vi "slscswitch Initialize.vi"(8 "error in (no error)":errorcluster, 9 "reset device (T)":bool, 11 "device":refnum<k21>) -> (0 "error out":errorcluster, 3 "SLSC Switch out":refnum<class "SLSC Switch.lvclass">)   [LabVIEW 2015, in "SLSC Switch.lvclass"]
uses:
  SLSC Switch.lvclass
  SLSC Switch.lvclass/SLSC Switch.ctl
  <vilib>/SLSC/Initialize Session without Resources.vi
  Route Manager/Route Manager.lvclass
  <vilib>/SLSC/SLSC.lvlib
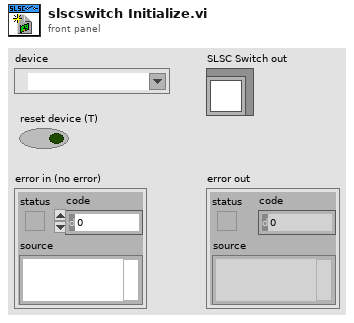
[diagram p1: front panel]
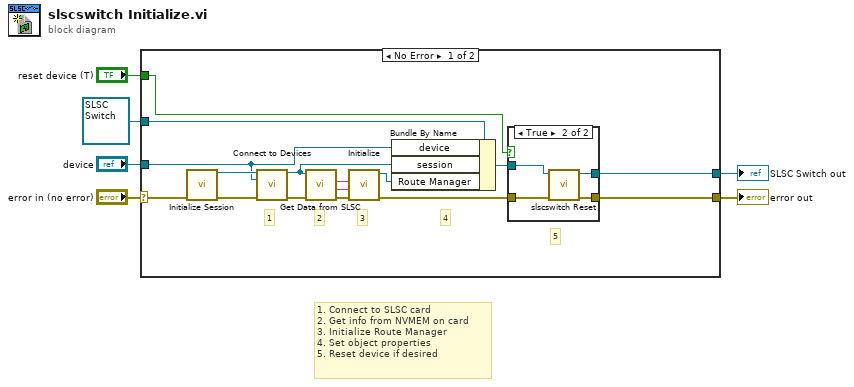
[diagram p0: block diagram]
diagram:
  # "1. Connect to SLSC card\n2. Get info from NVMEM on card\n3. Initialize Route Manager\n4. Set object properties\n5. Reset device if desired"
  n1 = case shown="No Error" "error in (no error)" {
    selector: "error in (no error)" -> [w10 w30]
    tunnel: [w13 w30] -> w5
    tunnel: [w14 w29] -> w3
    tunnel: refnum<class "SLSC Switch.lvclass"> refnum ("SLSC Switch in") -> [w20 w29]
    tunnel: "device" -> [w8 _]
    tunnel: "reset device (T)" -> [w17 _]
    frame No Error {
      # "5"
      # "4"
      # "3"
      # "2"
      # "1"
      n2 = call-poly <vilib>:"Initialize Session.vi"("error in (no error)"=w10) -> ("session out"=w12:refnum<k21>, "error out"=w11:errorcluster)  [unwired: 13 in]
      n3 = call <vilib>:"Connect to Devices.vi"("session in"=w12, "devices"=w8, "error in (no error)"=w11) -> ("session out"=w7:refnum<k21>, "error out"=w9:errorcluster)  [unwired: 11 in]
      n4 = call "Get Data from SLSC.vi"("error in (no error)"=w9, "session"=w7) -> ("error out"=w18:errorcluster, "top file info"=w21:string, "swt file info"=w22:string)  [unwired: 7 in]
      n5 = call "Initialize.vi"("error in (no error)"=w18, "top file info"=w21, "swt file info"=w22) -> ("error out"=w15:errorcluster, "Route Manager out"=w19:refnum<class "Route Manager.lvclass">)  [unwired: 7 in]
      n6 = Bundle By Name(cluster=w20, "device"=w8, "session"=w7, "Route Manager"=w19) -> (w16:refnum<class "SLSC Switch.lvclass">)
      n7 = case shown="True" w17 {
        tunnel: w16 -> [w24 w28]
        tunnel: w15 -> [w23 w27]
        tunnel: [w24 w26] -> w14
        tunnel: [w23 w25] -> w13
        frame False {
        }
        frame True {
          n8 = call "slscswitch Reset.vi"("error in (no error)"=w27, "SLSC Switch in"=w28) -> ("error out"=w25:errorcluster, "SLSC Switch out"=w26:refnum<class "SLSC Switch.lvclass">)  [unwired: 8 in]
        }
      }
    }
    frame Error {
    }
  }
  "error out" <- w5
  "SLSC Switch out" <- w3
